vi "HumanExecute.vi"(8 "error in (no error)":errorcluster) -> (0 "error out":errorcluster)   [LabVIEW 2023]
doc: "Execute for Human\n\ninput:\n error in (cluster)\n\noutput:\n error out (cluster)"
uses:
  <vilib>/Rock Robotics/WPI/Joystick/XBox Buttons Indexer.ctl
  <vilib>/Rock Robotics/WPI/Joystick/XBox Axes Indexer.ctl
  <vilib>/Rock Robotics/WPI/ThirdParty/JAS_Junk/TrajLib/VI/BoolCmd_Send_Internal.vi
  <vilib>/Rock Robotics/WPI/ThirdParty/JAS_Junk/TrajLib/VI/BoolCmd_ObtainQueue.vi
  HumanGlobal.vi
  <vilib>/Rock Robotics/Network Tables/NT Write String.vi
  <vilib>/Rock Robotics/WPI/ThirdParty/JAS_Junk/TrajLib/Trajectory_Library.lvlib
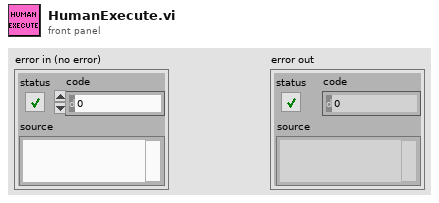
[diagram p1: front panel]
types:
  T1 = typedef "XBox Buttons Indexer.ctl" = enum16{"A", "B", "X", "Y", "Left Bumper", "Right Bumper", "Back", "Start", "Left Joystick", "Right Joystick"}
  T2 = typedef "XBox Axes Indexer.ctl" = enum16{"Left X", "Left Y", "Left Trigger", "Right Trigger", "Right X", "Right Y"}
  T3 = typedef "WPI_JoystickDevRef.ctl" = cluster{"Device":T4}
  T4 = typedef "WPI_JoystickDeviceEnum.ctl" = enum16{"USB 0", "USB 1", "USB 2", "USB 3", "USB 4", "USB 5"}
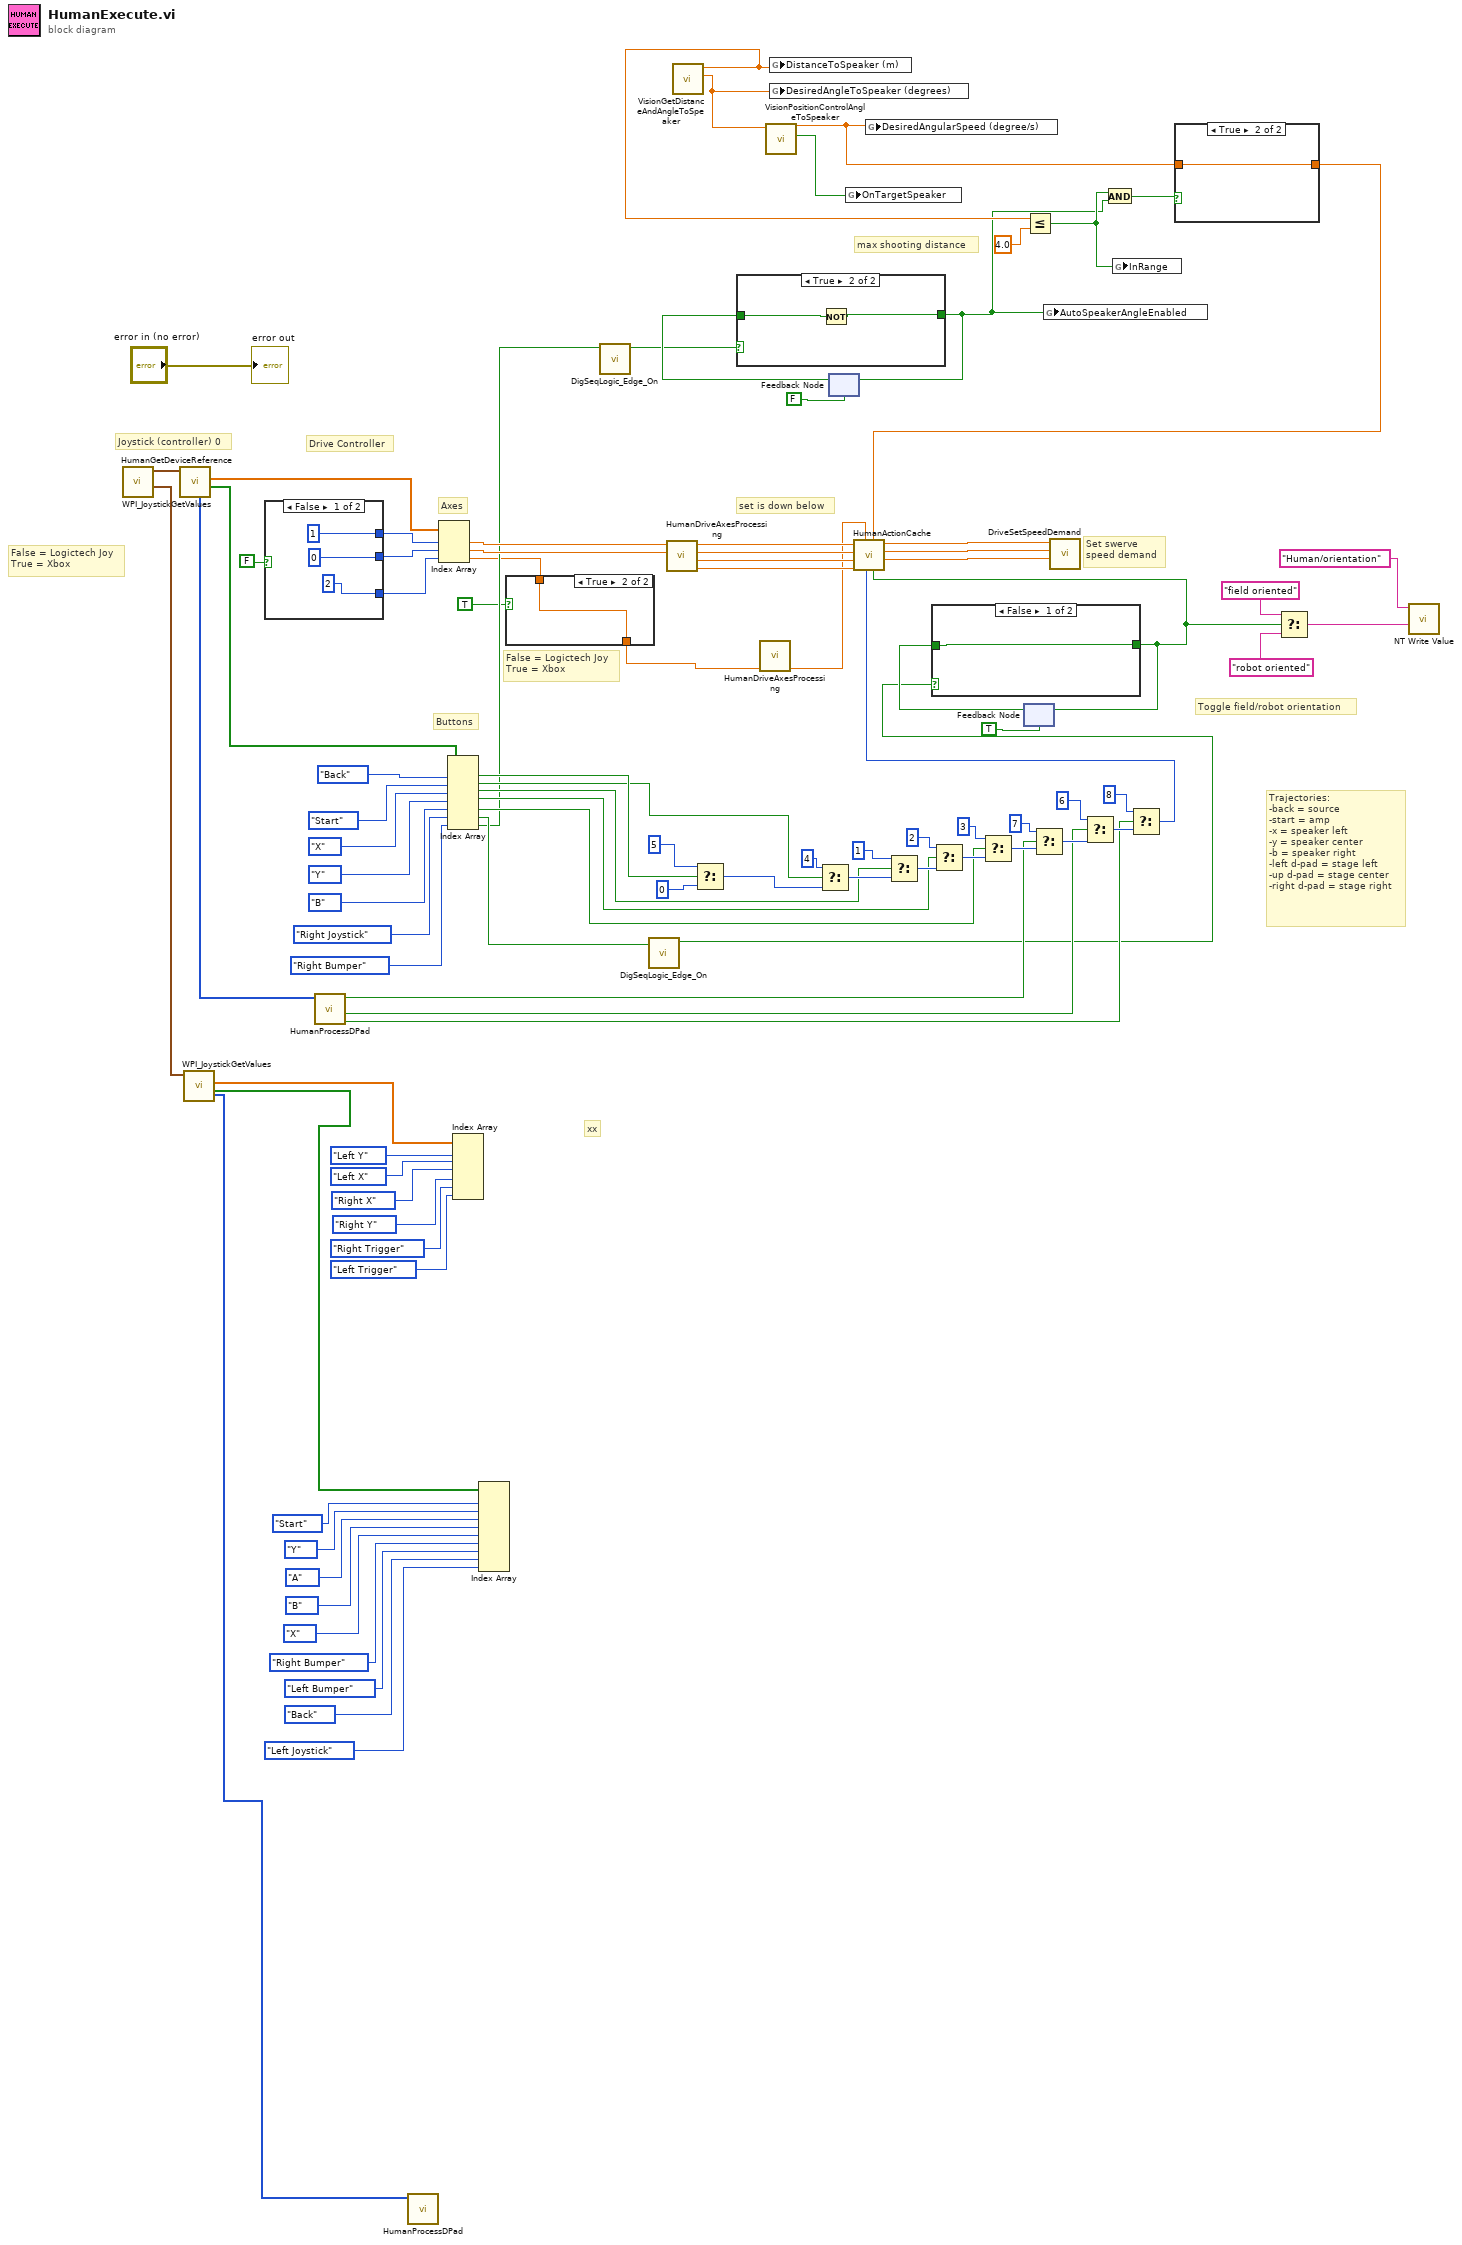
[diagram p0: block diagram]
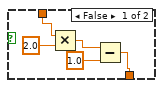
[diagram p2: hidden frame]
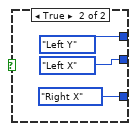
[diagram p3: hidden frame]
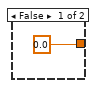
[diagram p5: hidden frame]
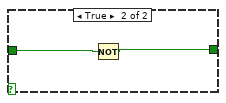
[diagram p6: hidden frame]
diagram:
  # "False = Logictech Joy\nTrue = Xbox"
  # "False = Logictech Joy\nTrue = Xbox"
  # "max shooting distance"
  # "Toggle field/robot orientation"
  # "xx"
  # "Trajectories:\n-back = source\n-start = amp\n-x = speaker left\n-y = speaker center\n-b = speaker right\n-left d-pad = stage left\n-up d-pad = stage center\n-right d-pad = stage right"
  # "Buttons"
  # "Axes"
  # "set is down below"
  # "Set swerve\nspeed demand"
  # "Joystick (controller) 0"
  # "Drive Controller"
  n1 = call "HumanGetDeviceReference.vi"() -> ("Aux Joy"=w79:T3, "Driver Joy"=w83:T3)  [unwired: 9 in, 1 out]
  n2 = call <vilib>:"WPI_JoystickGetValues.vi"("JoystickDevRef"=w83) -> ("Buttons"=w64:bool[], "Axes"=w65:dbl[], "POVs"=w92:i16[])  [unwired: 6 in, 2 out]
  n3 = call <vilib>:"WPI_JoystickGetValues.vi"("JoystickDevRef"=w79) -> ("Buttons"=w69:bool[], "Axes"=w78:dbl[], "POVs"=w57:i16[])  [unwired: 6 in, 2 out]
  n4 = case shown="False" FALSE {
    tunnel: [1 XBox_Axes_Indexer."Left Y" ("XBox Axes")] -> w95
    tunnel: [0 XBox_Axes_Indexer."Left X" ("XBox Axes")] -> w94
    tunnel: [2 XBox_Axes_Indexer."Right X" ("XBox Axes")] -> w58
    frame False {
    }
    frame True {
    }
  }
  n5 = call "HumanProcessDPad.vi"("POV"=w92) -> ("Right"=w40:bool, "Left"=w41:bool, "Up"=w42:bool)  [unwired: 7 in, 1 out]
  n6 = call "HumanProcessDPad.vi"("POV"=w57) -> ()  [unwired: 7 in, 4 out]
  n7 = Index Array(array=w65, index #1=w95, index #2=w94, index #3=w58) -> (element #1=w91:dbl, element #2=w90:dbl, element #3=w2:dbl)
  n8 = Index Array(array=w64, index #1=XBox_Buttons_Indexer."Back" ("Nothing"), index #2=XBox_Buttons_Indexer."Start" ("Nothing"), index #3=XBox_Buttons_Indexer."X" ("Nothing"), index #4=XBox_Buttons_Indexer."Y" ("Nothing"), index #5=XBox_Buttons_Indexer."B" ("Nothing"), index #6=XBox_Buttons_Indexer."Right Joystick" ("Nothing"), index #7=XBox_Buttons_Indexer."Right Bumper" ("Nothing")) -> (element #1=w56:bool, element #2=w46:bool, element #3=w45:bool, element #4=w44:bool, element #5=w43:bool, element #6=w30:bool, element #7=w10:bool)
  n9 = Index Array(array=w78, index #1=XBox_Axes_Indexer."Left Y" ("XBox Axes"), index #2=XBox_Axes_Indexer."Left X" ("XBox Axes"), index #3=XBox_Axes_Indexer."Right X" ("XBox Axes"), index #4=XBox_Axes_Indexer."Right Y" ("XBox Axes"), index #5=XBox_Axes_Indexer."Right Trigger" ("XBox Axes"), index #6=XBox_Axes_Indexer."Left Trigger" ("XBox Axes")) -> ()  [unwired: 6 out]
  n10 = Index Array "Index Array"(array=w69, index #1=XBox_Buttons_Indexer."Start" ("Nothing"), index #2=XBox_Buttons_Indexer."Y" ("OpenCloseClaw"), index #3=XBox_Buttons_Indexer."A" ("GrabberIn"), index #4=XBox_Buttons_Indexer."B" ("GrabberOut"), index #5=XBox_Buttons_Indexer."X" ("Nothing"), index #6=XBox_Buttons_Indexer."Right Bumper" ("Nothing"), index #7=XBox_Buttons_Indexer."Left Bumper" ("Nothing"), index #8=XBox_Buttons_Indexer."Back" ("Place Cone"), index #9=XBox_Buttons_Indexer."Left Joystick" ("Place Cone")) -> ()  [unwired: 9 out]
  n11 = case shown="True" TRUE {
    tunnel: [w103 w107] -> w3
    tunnel: w2 -> [w106 w107]
    frame False {
      n12 = Multiply(x=w106, y=2.0) -> (x*y=w104:dbl)
      n13 = Subtract(x=w104, y=1.0) -> (x-y=w103:dbl)
    }
    frame True {
    }
  }
  n14 = call <vilib>:"DigSeqLogic_Edge_On.vi"("Input"=w10) -> ("On Edge"=w11:bool)  [unwired: 10 in]
  n15 = call <vilib>:"DigSeqLogic_Edge_On.vi"("Input"=w30) -> ("On Edge"=w28:bool)  [unwired: 10 in]
  n16 = call "HumanDriveAxesProcessing.vi"("Left X"=w90, "Left Y"=w91) -> ("Right X"=w7:dbl, "Right Y"=w88:dbl, "Left X"=w89:dbl, "Left Y"=w87:dbl)  [unwired: 6 in]
  n17 = call "VisionGetDistanceAndAngleToSpeaker.vi"() -> ("DesiredAngle"=w21:dbl, "Distance"=w19:dbl)  [unwired: 10 in]
  n18 = Select(t=5, s=w56, f=0) -> (s? t:f=w53:i32)
  n19 = call "HumanDriveAxesProcessing.vi"("Right X"=w3) -> ("Right X"=w6:dbl)  [unwired: 7 in, 3 out]
  n20 = call "VisionPositionControlAngleToSpeaker.vi"("TargetAngle"=w21) -> ("OnTargetSpeaker"=w20:bool, "DesiredAngularSpeed (degree/s)"=w17:dbl)  [unwired: 9 in]
  n21 = global write "HumanGlobal.vi" "DistanceToSpeaker (m)"(w19) -> ()
  n22 = global write "HumanGlobal.vi" "DesiredAngleToSpeaker (degrees)"(w21) -> ()
  n23 = Select(t=4, s=w46, f=w53) -> (s? t:f=w52:i32)
  n24 = feedback #1(FALSE) -> (w13:bool)
  n25 = case shown="True" w11 {
    tunnel: w13 -> [w108 w110]
    tunnel: [w108 w109] -> w9
    frame False {
    }
    frame True {
      n26 = Not(x=w110) -> (.not. x?=w109:bool)
    }
  }
  n27 = feedback-in #1(w9) -> ()
  n28 = global write "HumanGlobal.vi" "OnTargetSpeaker"(w20) -> ()
  n29 = global write "HumanGlobal.vi" "DesiredAngularSpeed (degree/s)"(w17) -> ()
  n30 = Select(t=1, s=w45, f=w52) -> (s? t:f=w51:i32)
  n31 = Select(t=2, s=w44, f=w51) -> (s? t:f=w50:i32)
  n32 = Select(t=3, s=w43, f=w50) -> (s? t:f=w49:i32)
  n33 = feedback #2(TRUE) -> (w29:bool)
  n34 = case shown="False" w28 {
    tunnel: w29 -> [w111 w113]
    tunnel: [w111 w112] -> w26
    frame False {
    }
    frame True {
      n35 = Not(x=w113) -> (.not. x?=w112:bool)
    }
  }
  n36 = feedback-in #2(w26) -> ()
  n37 = Less Or Equal?(x=w19, y=4.0) -> (x <= y?=w16:bool)
  n38 = Select(t=7, s=w42, f=w49) -> (s? t:f=w48:i32)
  n39 = global write "HumanGlobal.vi" "AutoSpeakerAngleEnabled"(w9) -> ()
  n40 = Select(t=6, s=w41, f=w48) -> (s? t:f=w47:i32)
  n41 = And(x=w16, y=w9) -> (x .and. y?=w15:bool)
  n42 = global write "HumanGlobal.vi" "InRange"(w16) -> ()
  n43 = Select(t=8, s=w40, f=w47) -> (s? t:f=w32:i32)
  n44 = case shown="True" w15 {
    tunnel: w17 -> [_ w115]
    tunnel: [0.0 w115] -> w8
    frame False {
    }
    frame True {
    }
  }
  n45 = call "HumanActionCache.vi"("Enable Field Oriented Drive"=w26, "AutoSpeakerAngle"=w8, "State"=w32, "Rotation"=w6, "Right X"=w7, "Right Y"=w88, "Left X"=w89, "Left Y"=w87) -> ("AMotorDemand"=w86:dbl, "YMotorDemand"=w85:dbl, "XMotorDemand"=w84:dbl)  [unwired: 1 in]
  n46 = call "DriveSetSpeedDemand.vi"("ASpeedDemand (d/s)"=w86, "YSpeedDemand (ft/s)"=w85, "XSpeedDemand (ft/s)"=w84) -> ()  [unwired: 9 in]
  n47 = Select(t="field oriented", s=w26, f="robot oriented") -> (s? t:f=w23:string)
  n48 = call-poly <vilib>:"NT Write Value.vi"("value"=w23, "name"="Human/orientation") -> ()  [unwired: 9 in, 1 out]
  "error out" <- "error in (no error)"
